vi "Get nominal calibration coefficients from measured R0, RL.vi"(0 "R0 (ohm)":dbl=3.5000001778045013, 5 "RL (ohm)":dbl=0.4999997479390843, 7 "RG1 (ohm)":dbl=49.9, 9 "RG2 (ohm)":dbl=1600.0, 11 "RN (ohm)":dbl=4.32, 12 "I (A)":dbl=0.0001, 13 "alpha0 (/°C)":dbl=0.0036, 14 "T0 (°C)":dbl=20.0) -> (4 "Slope (°C / V)":dbl=25.12548, 8 "Intercept (°C)":dbl=45.39683000000001)   [LabVIEW 2020]
doc: "Calculate a probe's linear calibration coefficients from its measured R0 and RL.\nPN 05-NOV-2023."
panel:
  # "T = aV + b"
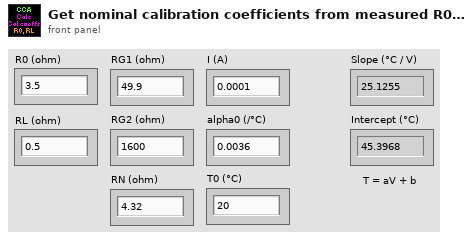
[diagram p1: front panel]
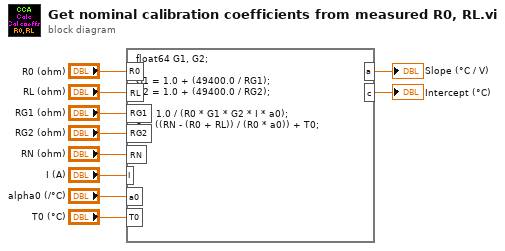
[diagram p0: block diagram]
diagram:
  n1 = formula code="float64 G1, G2;\n\nG1 = 1.0 + (49400.0 / RG1);\nG2 = 1.0 + (49400.0 / RG2);\n\na = 1.0 / (R0 * G1 * G2 * I * a0);\nc = ((RN - (R0 + RL)) / (R0 * a0)) + T0;"("RG1"="RG1 (ohm)", "RG2"="RG2 (ohm)", "RN"="RN (ohm)", "I"="I (A)", "a0"="alpha0 (/°C)", "R0"="R0 (ohm)", "RL"="RL (ohm)", "T0"="T0 (°C)") -> ("a"=→"Slope (°C / V)":dbl, "c"=→"Intercept (°C)":dbl)
